vi "CANdiGetters.vi"   [LabVIEW 2023]
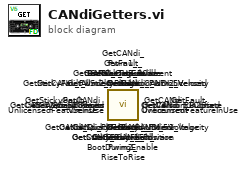
[diagram p0: block diagram]
diagram:
  n1 = call <vilib>:"GetStickyFault_CANDI_5V.vi"() -> ()  [unwired: 10 in, 2 out]
  n2 = call <vilib>:"GetFault_CANDI_5V.vi"() -> ()  [unwired: 10 in, 2 out]
  n3 = call <vilib>:"GetStickyFault_UnlicensedFeatureInUse.vi"() -> ()  [unwired: 10 in, 2 out]
  n4 = call <vilib>:"GetFault_UnlicensedFeatureInUse.vi"() -> ()  [unwired: 10 in, 2 out]
  n5 = call <vilib>:"GetStickyFault_BootDuringEnable.vi"() -> ()  [unwired: 10 in, 2 out]
  n6 = call <vilib>:"GetFault_BootDuringEnable.vi"() -> ()  [unwired: 10 in, 2 out]
  n7 = call <vilib>:"GetStickyFault_Undervoltage.vi"() -> ()  [unwired: 10 in, 2 out]
  n8 = call <vilib>:"GetFault_Undervoltage.vi"() -> ()  [unwired: 10 in, 2 out]
  n9 = call <vilib>:"GetStickyFault_Hardware.vi"() -> ()  [unwired: 10 in, 2 out]
  n10 = call <vilib>:"GetFault_Hardware.vi"() -> ()  [unwired: 10 in, 2 out]
  n11 = call <vilib>:"GetCANdi_S2Closed.vi"() -> ()  [unwired: 10 in, 2 out]
  n12 = call <vilib>:"GetCANdi_S1Closed.vi"() -> ()  [unwired: 10 in, 2 out]
  n13 = call <vilib>:"GetCANdi_QuadVelocity.vi"() -> ()  [unwired: 10 in, 2 out]
  n14 = call <vilib>:"GetCANdi_Pwm2_Velocity.vi"() -> ()  [unwired: 10 in, 2 out]
  n15 = call <vilib>:"GetCANdi_OutputCurrent.vi"() -> ()  [unwired: 10 in, 2 out]
  n16 = call <vilib>:"GetCANdi_VSense.vi"() -> ()  [unwired: 10 in, 2 out]
  n17 = call <vilib>:"GetCANdi_Overcurrent.vi"() -> ()  [unwired: 10 in, 2 out]
  n18 = call <vilib>:"GetCANdi_Pwm2_Position.vi"() -> ()  [unwired: 10 in, 2 out]
  n19 = call <vilib>:"GetCANdi_Pwm2_RiseToRise.vi"() -> ()  [unwired: 10 in, 2 out]
  n20 = call <vilib>:"GetCANdi_Pwm1_Velocity.vi"() -> ()  [unwired: 10 in, 2 out]
  n21 = call <vilib>:"GetCANdi_Pwm1_Position.vi"() -> ()  [unwired: 10 in, 2 out]
  n22 = call <vilib>:"GetCANdi_Pwm1_RiseToRise.vi"() -> ()  [unwired: 10 in, 2 out]
  n23 = call <vilib>:"GetCANdi_QuadPosition.vi"() -> ()  [unwired: 10 in, 2 out]
  n24 = call <vilib>:"GetCANdi_Pin2State.vi"() -> ()  [unwired: 10 in, 2 out]
  n25 = call <vilib>:"GetCANdi_Pin1State.vi"() -> ()  [unwired: 10 in, 2 out]
  n26 = call <vilib>:"GetVersion_IsProLicensed.vi"() -> ()  [unwired: 10 in, 2 out]
  n27 = call <vilib>:"GetAllStickyFaults.vi"() -> ()  [unwired: 10 in, 2 out]
  n28 = call <vilib>:"GetAllFaults.vi"() -> ()  [unwired: 10 in, 2 out]
  n29 = call <vilib>:"GetVersion_Full.vi"() -> ()  [unwired: 10 in, 2 out]
  n30 = call <vilib>:"GetVersion_Build.vi"() -> ()  [unwired: 10 in, 2 out]
  n31 = call <vilib>:"GetVersion_Bugfix.vi"() -> ()  [unwired: 10 in, 2 out]
  n32 = call <vilib>:"GetVersion_Minor.vi"() -> ()  [unwired: 10 in, 2 out]
  n33 = call <vilib>:"GetVersion_Major.vi"() -> ()  [unwired: 10 in, 2 out]
